vi "Create Pattern Script(DataCapture).vi"(7 "Opcode":string, 8 "error in (no error)":errorcluster, 9 "Num of Cycles":i8, 10 "BurstLength":T1, 11 "BML Pattern Creater in":refnum<class "BML Pattern Creater.lvclass">) -> (0 "error out":errorcluster, 2 "String":string, 3 "BML Pattern Creater out":refnum<class "BML Pattern Creater.lvclass">)   [LabVIEW 2018, in "BML Pattern Creater.lvlib" / "BML Pattern Creater.lvclass"]
uses:
  BML Pattern Creater.lvclass
  Ctls/Burst Length.ctl
  Interfaces/Protocol Interface.lvlibp/Interfaces/Protocol Interface/Pin State.ctl
  Interfaces/Protocol Interface.lvlibp/Interfaces/Protocol Interface/Protocol Interface.lvclass
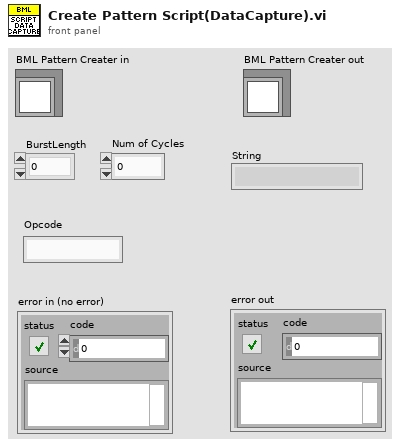
[diagram p1: front panel]
types:
  T1 = typedef "Burst Length.ctl" = enum8{"0", "2", "3", "4", "5", "8", "16", "32"}
  T2 = typedef "Protocol Interface.lvlibp/Protocol Interface.lvclass/Pin State.ctl" = enum16{"0", "1", "L", "H", "X", "V", "D", "M"}
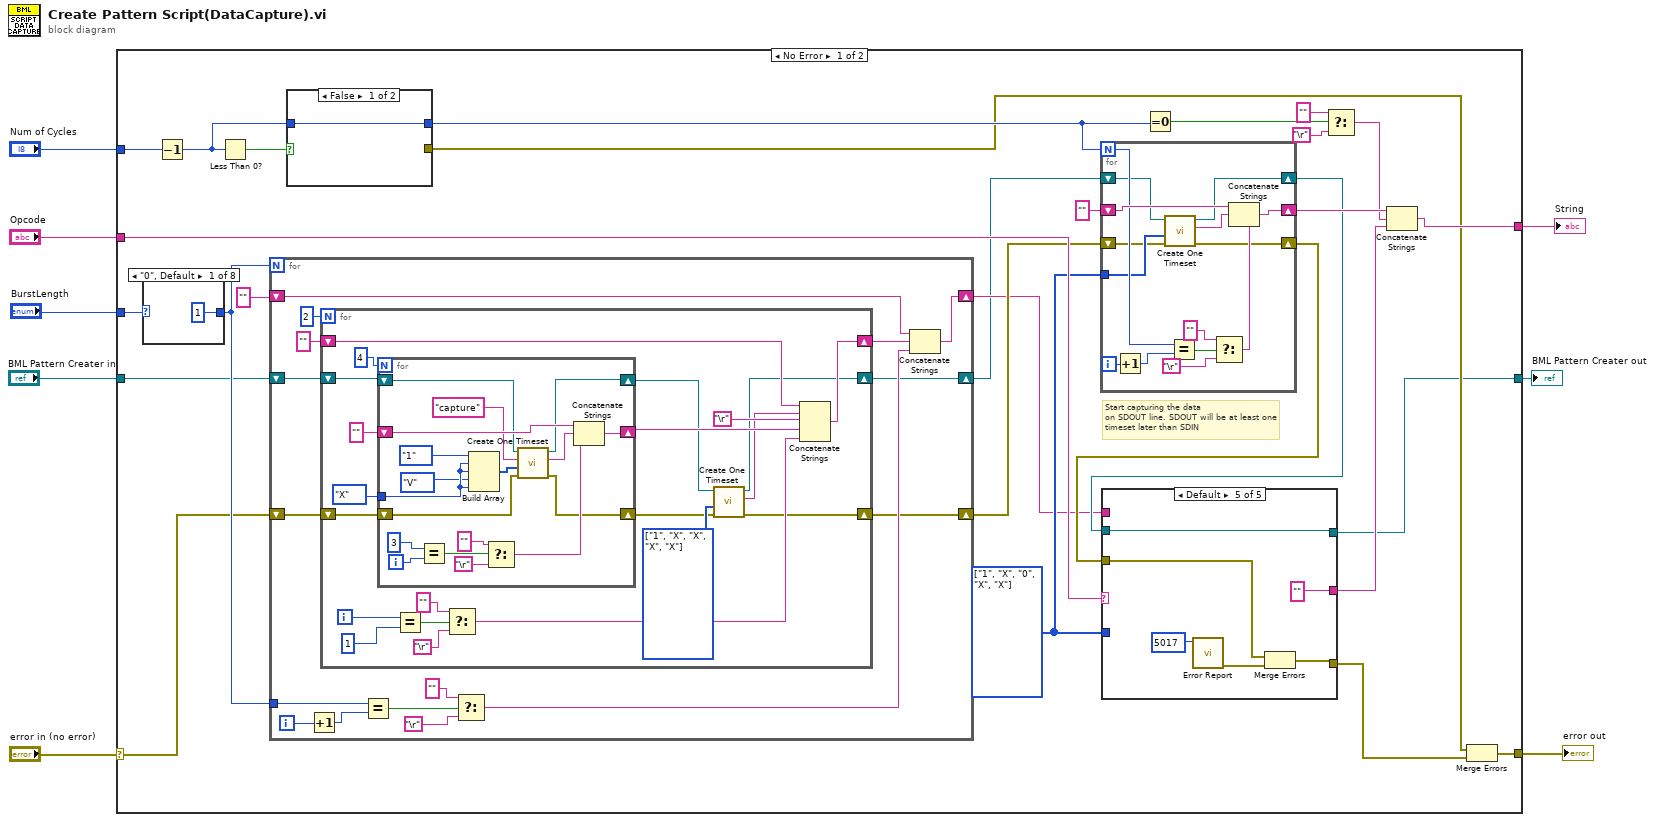
[diagram p0: block diagram]
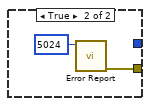
[diagram p2: hidden frame]
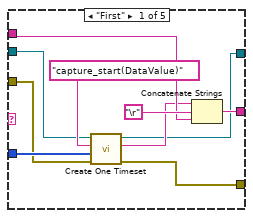
[diagram p3: hidden frame]
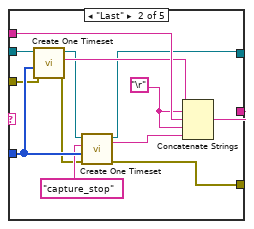
[diagram p4: hidden frame]
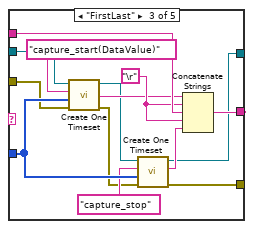
[diagram p5: hidden frame]
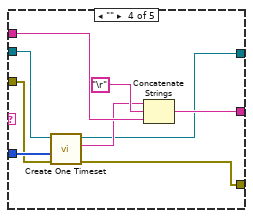
[diagram p6: hidden frame]
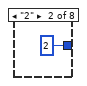
[diagram p7: hidden frame]
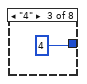
[diagram p8: hidden frame]
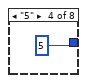
[diagram p9: hidden frame]
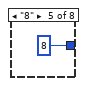
[diagram p10: hidden frame]
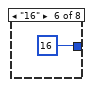
[diagram p11: hidden frame]
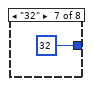
[diagram p12: hidden frame]
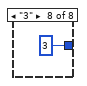
[diagram p13: hidden frame]
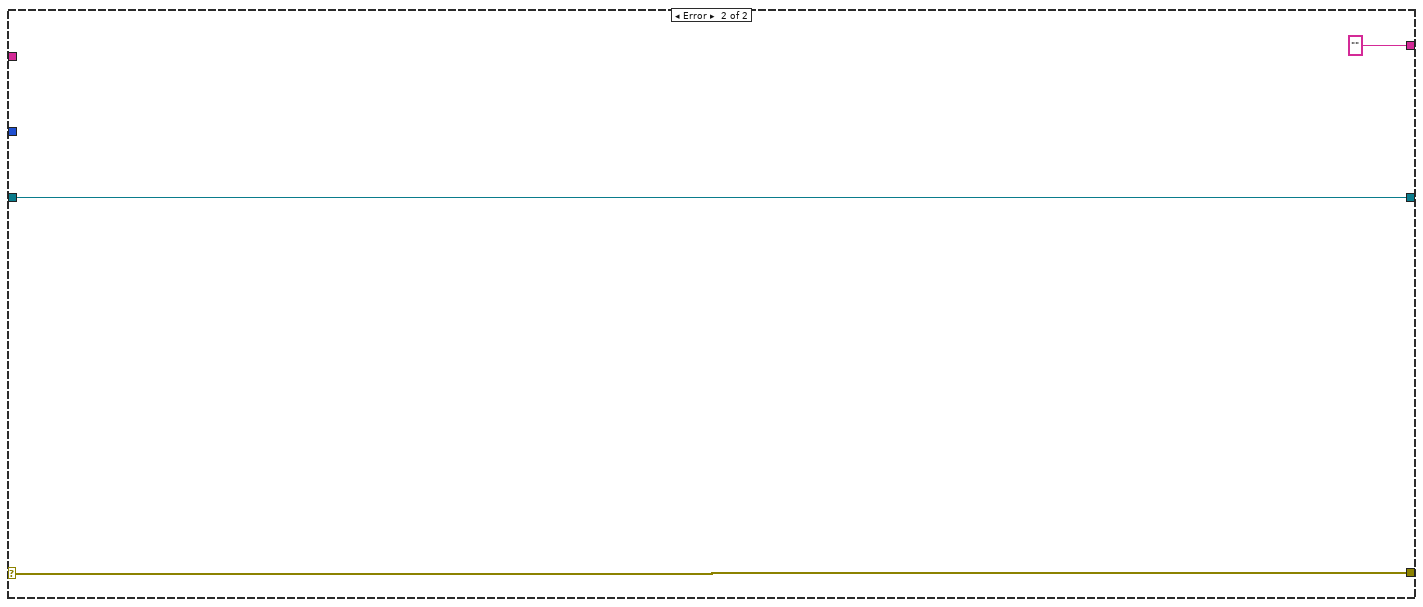
[diagram p14: hidden frame]
diagram:
  n1 = case shown="No Error" "error in (no error)" {
    selector: "error in (no error)" -> [w14 w171]
    tunnel: [w19 ""] -> w7
    tunnel: [w32 w171] -> w6
    tunnel: "BurstLength" -> [w35 _]
    tunnel: "Opcode" -> [w33 _]
    tunnel: "Num of Cycles" -> [w30 _]
    tunnel: [w10 w170] -> w1
    tunnel: "BML Pattern Creater in" -> [w9 w170]
    frame No Error {
      w17 = T2[] [enum."1", enum."X", enum."0", enum."X", enum."X"] items=["0", "1", "L", "H", "X", "V", "D", "M"]
      # "Start capturing the data\non SDOUT line. SDOUT will be at least one \ntimeset later than SDIN"
      n2 = case shown="\"0\", Default" w35 {
        tunnel: [1 ("y") 2 ("y") 4 ("y") 5 ("y") 8 ("y") 16 ("y") 32 ("y") 3 ("y")] -> w34
        frame "0", Default {
        }
        frame "2" {
        }
        frame "4" {
        }
        frame "5" {
        }
        frame "8" {
        }
        frame "16" {
        }
        frame "32" {
        }
        frame "3" {
        }
      }
      n3 = Decrement(x=w30) -> (x-1=w27:i8)
      n4 = Less Than 0?(x=w27) -> (x < 0?=w28:bool)
      n5 = for {
        N: w34 -> [_]
        shift-right: [w121] -> w12
        shift-left: "" -> [w120]
        tunnel: w34 -> [w119]
        shift-right: [w118] -> w13
        shift-left: w14 -> [w117]
        shift-right: [w116] -> w11
        shift-left: w9 -> [w115]
        i -> [w128]
        n6 = Increment(x=w128) -> (x+1=w127:i32)
        n7 = for {
          N: 2 -> [_]
          shift-right: [w143] -> w123
          shift-left: "" -> [w141]
          shift-right: [w134] -> w118
          shift-left: w117 -> [w133]
          shift-right: [w132] -> w116
          shift-left: w115 -> [w131]
          i -> [w150]
          w138 = T2[] [enum."1", enum."X", enum."X", enum."X", enum."X"] items=["0", "1", "L", "H", "X", "V", "D", "M"]
          n8 = for {
            N: 4 -> [_]
            shift-right: [w164] -> w145
            shift-left: "" -> [w161]
            tunnel: Pin_State."X" ("PinState") -> [w162]
            shift-right: [w155] -> w136
            shift-left: w131 -> [w154]
            shift-right: [w153] -> w135
            shift-left: w133 -> [w152]
            i -> [w169]
            n9 = Equal?(x=3, y=w169) -> (x = y?=w167:bool)
            n10 = Build Array(Pin_State."1" ("PinState"), w162, w162, Pin_State."V" ("PinState"), w162) -> (w159:T2[])
            n11 = Select(t="", s=w167, f="\r") -> (s? t:f=w163:string)
            n12 = call-dynamic "Create One Timeset.vi"("error in (no error)"=w152, "Pin State"=w159, "opcode"="capture", "BML Pattern Creater in"=w154) -> ("error out"=w153:errorcluster, "string out"=w158:string, "BML Pattern Creater out"=w155:refnum<class "BML Pattern Creater.lvclass">)  [unwired: 5 in]
            n13 = Concatenate Strings(w161, w158, w163) -> (w164:string)
          }
          n14 = Equal?(x=w150, y=1) -> (x = y?=w148:bool)
          n15 = Select(t="", s=w148, f="\r") -> (s? t:f=w144:string)
          n16 = call-dynamic "Create One Timeset.vi"("error in (no error)"=w135, "Pin State"=w138, "BML Pattern Creater in"=w136) -> ("error out"=w134:errorcluster, "string out"=w139:string, "BML Pattern Creater out"=w132:refnum<class "BML Pattern Creater.lvclass">)  [unwired: 6 in]
          n17 = Concatenate Strings(w141, w139, "\r", w145, w144) -> (w143:string)
        }
        n18 = Equal?(x=w119, y=w127) -> (x = y?=w124:bool)
        n19 = Select(t="", s=w124, f="\r") -> (s? t:f=w122:string)
        n20 = Concatenate Strings(w120, w123, w122) -> (w121:string)
      }
      n21 = case shown="False" w28 {
        tunnel: w27 -> [w37 _]
        tunnel: [w37 _] -> w25
        tunnel: [_ w38] -> w18
        frame False {
        }
        frame True {
          n22 = call "Error Report.vi"("Error Code"=i16 5024) -> ("error out"=w38:errorcluster)  [unwired: 10 in]
        }
      }
      n23 = for {
        N: w25 -> [w45]
        shift-right: [w54] -> w26
        shift-left: "" -> [w53]
        tunnel: w17 -> [w44]
        shift-right: [w43] -> w16
        shift-left: w13 -> [w42]
        shift-right: [w41] -> w15
        shift-left: w11 -> [w40]
        i -> [w48]
        n24 = Increment(x=w48) -> (x+1=w52:i32)
        n25 = call-dynamic "Create One Timeset.vi"("error in (no error)"=w42, "Pin State"=w44, "BML Pattern Creater in"=w40) -> ("error out"=w43:errorcluster, "string out"=w46:string, "BML Pattern Creater out"=w41:refnum<class "BML Pattern Creater.lvclass">)  [unwired: 6 in]
        n26 = Equal?(x=w45, y=w52) -> (x = y?=w49:bool)
        n27 = Select(t="", s=w49, f="\r") -> (s? t:f=w47:string)
        n28 = Concatenate Strings(w53, w46, w47) -> (w54:string)
      }
      n29 = case shown="Default" w33 {
        tunnel: w17 -> [w61 w72 w85 w97 _]
        tunnel: w12 -> [w63 w77 w91 w100 _]
        tunnel: [w62 w76 w90 w99 ""] -> w20
        tunnel: [w58 w68 w81 w95 w102] -> w31
        tunnel: w16 -> [w56 w67 w79 w92 w103]
        tunnel: w15 -> [w57 w66 w80 w94 w104]
        tunnel: [w55 w65 w78 w93 w104] -> w10
        frame "First" {
          n30 = call-dynamic "Create One Timeset.vi"("error in (no error)"=w56, "Pin State"=w61, "opcode"="capture_start(DataValue)", "BML Pattern Creater in"=w57) -> ("error out"=w58:errorcluster, "string out"=w60:string, "BML Pattern Creater out"=w55:refnum<class "BML Pattern Creater.lvclass">)  [unwired: 5 in]
          n31 = Concatenate Strings(w60, "\r", w63) -> (w62:string)
        }
        frame "Last" {
          w75 = "\r"
          n32 = call-dynamic "Create One Timeset.vi"("error in (no error)"=w67, "Pin State"=w72, "BML Pattern Creater in"=w66) -> ("error out"=w70:errorcluster, "string out"=w74:string, "BML Pattern Creater out"=w69:refnum<class "BML Pattern Creater.lvclass">)  [unwired: 6 in]
          n33 = call-dynamic "Create One Timeset.vi"("error in (no error)"=w70, "Pin State"=w72, "opcode"="capture_stop", "BML Pattern Creater in"=w69) -> ("error out"=w68:errorcluster, "string out"=w73:string, "BML Pattern Creater out"=w65:refnum<class "BML Pattern Creater.lvclass">)  [unwired: 5 in]
          n34 = Concatenate Strings(w74, w75, w77, w75, w73) -> (w76:string)
        }
        frame "FirstLast" {
          w89 = "\r"
          n35 = call-dynamic "Create One Timeset.vi"("error in (no error)"=w79, "Pin State"=w85, "opcode"="capture_start(DataValue)", "BML Pattern Creater in"=w80) -> ("error out"=w83:errorcluster, "string out"=w88:string, "BML Pattern Creater out"=w82:refnum<class "BML Pattern Creater.lvclass">)  [unwired: 5 in]
          n36 = call-dynamic "Create One Timeset.vi"("error in (no error)"=w83, "Pin State"=w85, "opcode"="capture_stop", "BML Pattern Creater in"=w82) -> ("error out"=w81:errorcluster, "string out"=w86:string, "BML Pattern Creater out"=w78:refnum<class "BML Pattern Creater.lvclass">)  [unwired: 5 in]
          n37 = Concatenate Strings(w88, w89, w91, w89, w86) -> (w90:string)
        }
        frame "" {
          n38 = call-dynamic "Create One Timeset.vi"("error in (no error)"=w92, "Pin State"=w97, "BML Pattern Creater in"=w94) -> ("error out"=w95:errorcluster, "string out"=w96:string, "BML Pattern Creater out"=w93:refnum<class "BML Pattern Creater.lvclass">)  [unwired: 6 in]
          n39 = Concatenate Strings(w96, "\r", w100) -> (w99:string)
        }
        frame Default {
          n40 = call "Error Report.vi"("Error Code"=i16 5017) -> ("error out"=w101:errorcluster)  [unwired: 10 in]
          n41 = Merge Errors(w103, w101) -> (w102:errorcluster)
        }
      }
      n42 = Equal To 0?(x=w25) -> (x = 0?=w24:bool)
      n43 = Select(t="", s=w24, f="\r") -> (s? t:f=w21:string)
      n44 = Concatenate Strings(w26, w21, w20) -> (w19:string)
      n45 = Merge Errors(w18, w31) -> (w32:errorcluster)
    }
    frame Error {
    }
  }
  "String" <- w7
  "error out" <- w6
  "BML Pattern Creater out" <- w1
